vi "GenerateArm.vi"(0 "Text In":string, 1 "Arm Width":dbl=0.03 format="%.2f", 2 "Frame Start":T1={"nx"=1.0, "ny"=0.0, "nz"=0.0, "nw"=0.0, "ox"=0.0, "oy"=1.0, "oz"=0.0, "ow"=0.0, "ax"=0.0, "ay"=0.0, "az"=1.0, "aw"=0.0, "Px"=0.0, "Py"=0.0, "Pz"=0.0, "Pw"=1.0} {"Pw" format="%.2f"; "Pz" format="%.2f"; "Py" format="%.2f"; "Px" format="%.2f"; "aw" format="%.2f"; "az" format="%.2f"; "ay" format="%.2f"; "ax" format="%.2f"; "ow" format="%.2f"; "nw" format="%.2f"; "oz" format="%.2f"; "oy" format="%.2f"; "ox" format="%.2f"; "nz" format="%.2f"; "ny" format="%.2f"; "nx" format="%.2f"}, 3 "Frame End":T1={"nx"=1.0, "ny"=0.0, "nz"=0.0, "nw"=0.0, "ox"=0.0, "oy"=1.0, "oz"=0.0, "ow"=0.0, "ax"=0.0, "ay"=0.0, "az"=1.0, "aw"=0.0, "Px"=0.0, "Py"=0.0, "Pz"=0.0, "Pw"=1.0} {"Pw" format="%.2f"; "Pz" format="%.2f"; "Py" format="%.2f"; "Px" format="%.2f"; "aw" format="%.2f"; "az" format="%.2f"; "ay" format="%.2f"; "ax" format="%.2f"; "ow" format="%.2f"; "nw" format="%.2f"; "oz" format="%.2f"; "oy" format="%.2f"; "ox" format="%.2f"; "nz" format="%.2f"; "ny" format="%.2f"; "nx" format="%.2f"}, 4 "Color":u32(colorbox)=13421772) -> (5 "Text Out":string="Shape {\nappearance Appearance {\nmaterial Material {\nemissiveColor 0.80 0.80 0.80\n}\n}\ngeometry IndexedLineSet {\ncoord Coordinate {\npoint [\n0.00 0.00 0.00,0.00 0.00 0.00]}\ncoordIndex [0, 1\r]}}")   [LabVIEW 2010]
uses:
  ReferenceFrame.ctl
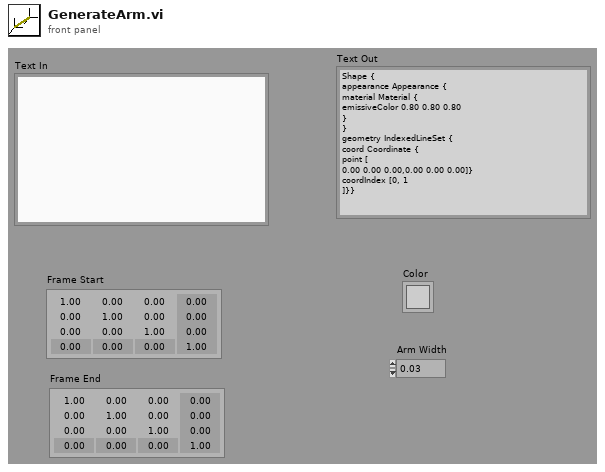
[diagram p1: front panel]
types:
  T1 = typedef "ReferenceFrame.ctl" = cluster{"nx":dbl, "ny":dbl, "nz":dbl, "nw":dbl, "ox":dbl, "oy":dbl, "oz":dbl, "ow":dbl, "ax":dbl, "ay":dbl, "az":dbl, "aw":dbl, "Px":dbl, "Py":dbl, "Pz":dbl, "Pw":dbl}
  T2 = cluster{"X":sgl, "Y":sgl, "Z":sgl, "roll":sgl, "pitch":sgl, "yaw":sgl}
  T3 = typedef "SinglePoint.ctl" = cluster{"X":dbl, "Y":dbl, "Z":dbl, "w":dbl}
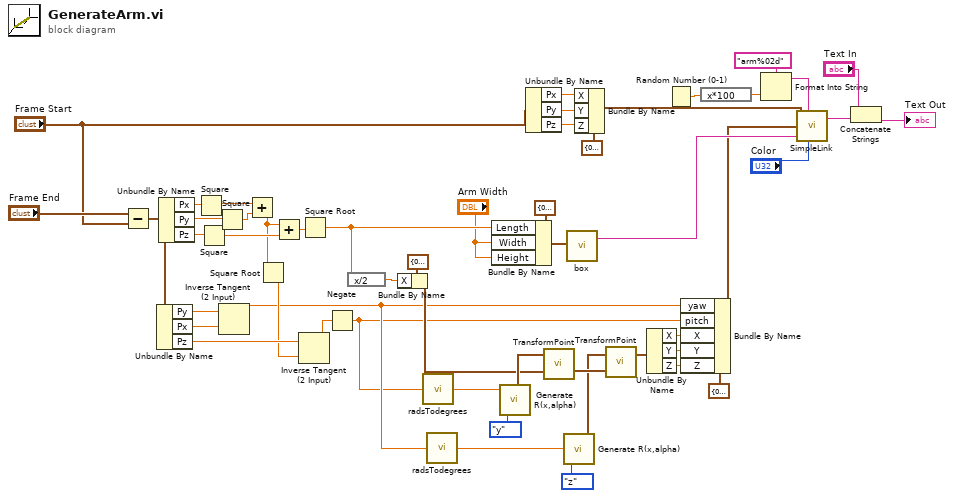
[diagram p0: block diagram]
diagram:
  n1 = Subtract(x="Frame End", y="Frame Start") -> (x-y=w35:T1)
  n2 = Unbundle By Name(w35) -> ("Py"=w34:dbl, "Px"=w33:dbl, "Pz"=w28:dbl)
  n3 = Unbundle By Name(w35) -> ("Px"=w41:dbl, "Py"=w42:dbl, "Pz"=w38:dbl)
  n4 = Square(x=w41) -> (x^2=w39:dbl)
  n5 = Square(x=w38) -> (x^2=w37:dbl)
  n6 = Square(x=w42) -> (x^2=w40:dbl)
  n7 = Inverse Tangent (2 Input)(1:w33, 2:w34) -> (0:w3:dbl)
  n8 = Add(x=w39, y=w40) -> (x+y=w27:dbl)
  n9 = Square Root(x=w27) -> (sqrt(x)=w26:dbl)
  n10 = Add(x=w27, y=w37) -> (x+y=w36:dbl)
  n11 = Inverse Tangent (2 Input)(1:w26, 2:w28) -> (0:w25:dbl)
  n12 = Square Root(x=w36) -> (sqrt(x)=w30:dbl)
  n13 = Negate(x=w25) -> (-x=w2:dbl)
  n14 = expression code="x/2"(w30) -> (w13:dbl)
  n15 = Bundle By Name(cluster=cluster{"X":dbl, "Y":dbl, "Z":dbl, "w":dbl} {"X"=0.0, "Y"=0.0, "Z"=0.0, "w"=0.0} ("P"), "X"=w13) -> (w4:cluster{"X":dbl, "Y":dbl, "Z":dbl, "w":dbl})
  n16 = call "radsTodegrees.vi"("Radians"=w2) -> ("Degrees"=w14:dbl)
  n17 = call "radsTodegrees.vi"("Radians"=w3) -> ("Degrees"=w12:dbl)
  n18 = Bundle By Name(cluster=cluster{"Length":sgl, "Width":sgl, "Height":sgl} {"Length"=0.6, "Width"=0.02, "Height"=0.02} ("Box"), "Length"=w30, "Width"="Arm Width", "Height"="Arm Width") -> (w24:cluster{"Length":sgl, "Width":sgl, "Height":sgl})
  n19 = call "Generate R(x,alpha).vi"("Axis"=enum16{"x", "y", "z"}."y", "Angle (degrees)"=w14) -> ("Final Frame"=w6:T1)  [unwired: 1 in]
  n20 = Unbundle By Name("Frame Start") -> ("Px"=w23:dbl, "Py"=w22:dbl, "Pz"=w21:dbl)
  n21 = call "TransformPoint.vi"("P"=w4, "A"=w6) -> ("AxP"=w9:T3)  [unwired: 1 out]
  n22 = call "Generate R(x,alpha).vi"("Axis"=enum16{"x", "y", "z"}."z", "Angle (degrees)"=w12) -> ("Final Frame"=w5:T1)  [unwired: 1 in]
  n23 = call "box.vi"("Box"=w24) -> ("urdf out"=w50:string)  [unwired: 3 in]
  n24 = Bundle By Name(cluster=T2 {"X"=0.0, "Y"=0.0, "Z"=0.0, "roll"=0.0, "pitch"=0.0, "yaw"=0.0} ("Pose"), "X"=w23, "Y"=w22, "Z"=w21) -> (w11:T2)
  n25 = call "TransformPoint.vi"("P"=w9, "A"=w5) -> ("AxP"=w7:T3)  [unwired: 1 out]
  n26 = Unbundle By Name(w7) -> ("X"=w15:dbl, "Y"=w16:dbl, "Z"=w17:dbl)
  n27 = Random Number (0-1)() -> (number: 0 to 1=w45:dbl)
  n28 = Bundle By Name(cluster=T2 {"X"=0.0, "Y"=0.0, "Z"=0.0, "roll"=0.0, "pitch"=0.0, "yaw"=0.0} ("Pose"), "yaw"=w3, "pitch"=w2, "X"=w15, "Y"=w16, "Z"=w17) -> (w10:T2)
  n29 = expression code="x*100"(w45) -> (w46:dbl)
  n30 = Format Into String(format string="arm%02d" ("Name"), w46) -> (resulting string=w47:string)  [unwired: 2 in, 1 out]
  n31 = call "SimpleLink.vi"("Geometry"=w11, "Name"=w47, "origin"=w10, "mass"=w50, "link color"="Color") -> ("link out"=w44:string)  [unwired: 1 in]
  n32 = Concatenate Strings("Text In", w44) -> (→"Text Out":string)
